vi "Climbing to Second Level.vi"(0 "close arms":bool, 1 "Second Preperation":bool, 2 "pull wire":bool, 3 "Open arms":bool, 4 "Abandon":bool) -> (5 "Prep 2":bool)   [LabVIEW 2012]
uses:
  <vilib>/Rock Robotics/WPI/PWM/Servo/WPI_ServoDeviceRef.ctl
  <vilib>/Rock Robotics/SystemInterfaces/Typedef/FPGA_TypedefDigitalModule.ctl
  <vilib>/Rock Robotics/SystemInterfaces/DIO/FPGA_DIOPWMChannel.ctl
  <vilib>/Rock Robotics/WPI/PWM/WPI_PWMDeadband.ctl
  <vilib>/Rock Robotics/WPI/MotorControl/WPI_MotorControlDeviceRef.ctl
  <vilib>/Rock Robotics/WPI/CAN/Jaguar/SubVIs/WPI_CANJaguar_ControlMode.ctl
  <vilib>/Rock Robotics/WPI/PWM/WPI_PWMTransform_ConPane.ctl
  BotStatus.vi
  Motors Values.vi
panel:
  out "cannenet vbus":dbl
  in  "Gyro Angle [degrees]":dbl
  in  "Analog Encoder Rotations [rotations]":dbl
  in  "distance of telescopit per one encoder rotation [m/rotations]":dbl
  in  "distance MAX of telescopit [m]":dbl
  in  "Telescopit Angle offset from horizon [degrees]":dbl
  in  "Telescopit set point Angle [degrees]":dbl
  in  "Start Climbing":bool
  out "telescopic vbus":dbl
  in  "Climbing":bool
  out "Telescopic Arms":dbl
  out "Canenet":dbl
  out "Climbing Enabled?":bool
  in  "Stop Climbing Override":bool
  in  "MotorControlDevRef 2":T1={"DeviceStatus"={"status"=FALSE, "code"=0, "source"=""}, "Type"=enum."PWM", "PWM"={"Digital Module"=enum."Digital Module 1", "PWM Channel"=enum."Invalid", "DeadBand"={"Name"="", "maxPositivePwm"=0, "minPositivePwm"=0, "centerPwm"=0, "maxNegativePwm"=0, "minNegativePwm"=0, "angularRange"=0}}, "CAN"={"Device Number"=0, "Control Mode"=enum."Percent VBus", "Semaphore"=refnum, "Max Vout"=12.0}, "Invert"=FALSE, "TransformRef"=refnum, "InvTransformRef"=refnum}
  in  "MotorControlDevRef 1":T1={"DeviceStatus"={"status"=FALSE, "code"=0, "source"=""}, "Type"=enum."PWM", "PWM"={"Digital Module"=enum."Digital Module 1", "PWM Channel"=enum."Invalid", "DeadBand"={"Name"="", "maxPositivePwm"=0, "minPositivePwm"=0, "centerPwm"=0, "maxNegativePwm"=0, "minNegativePwm"=0, "angularRange"=0}}, "CAN"={"Device Number"=0, "Control Mode"=enum."Percent VBus", "Semaphore"=refnum, "Max Vout"=12.0}, "Invert"=FALSE, "TransformRef"=refnum, "InvTransformRef"=refnum}
  in  "Climbing_ServoDeviceRef":T8={"DeviceStatus"={"status"=FALSE, "code"=0, "source"=""}, "Digital Module"=enum."Digital Module 1", "PWM Channel"=enum."Invalid", "DeadBand"={"Name"="", "maxPositivePwm"=0, "minPositivePwm"=0, "centerPwm"=0, "maxNegativePwm"=0, "minNegativePwm"=0, "angularRange"=0}}
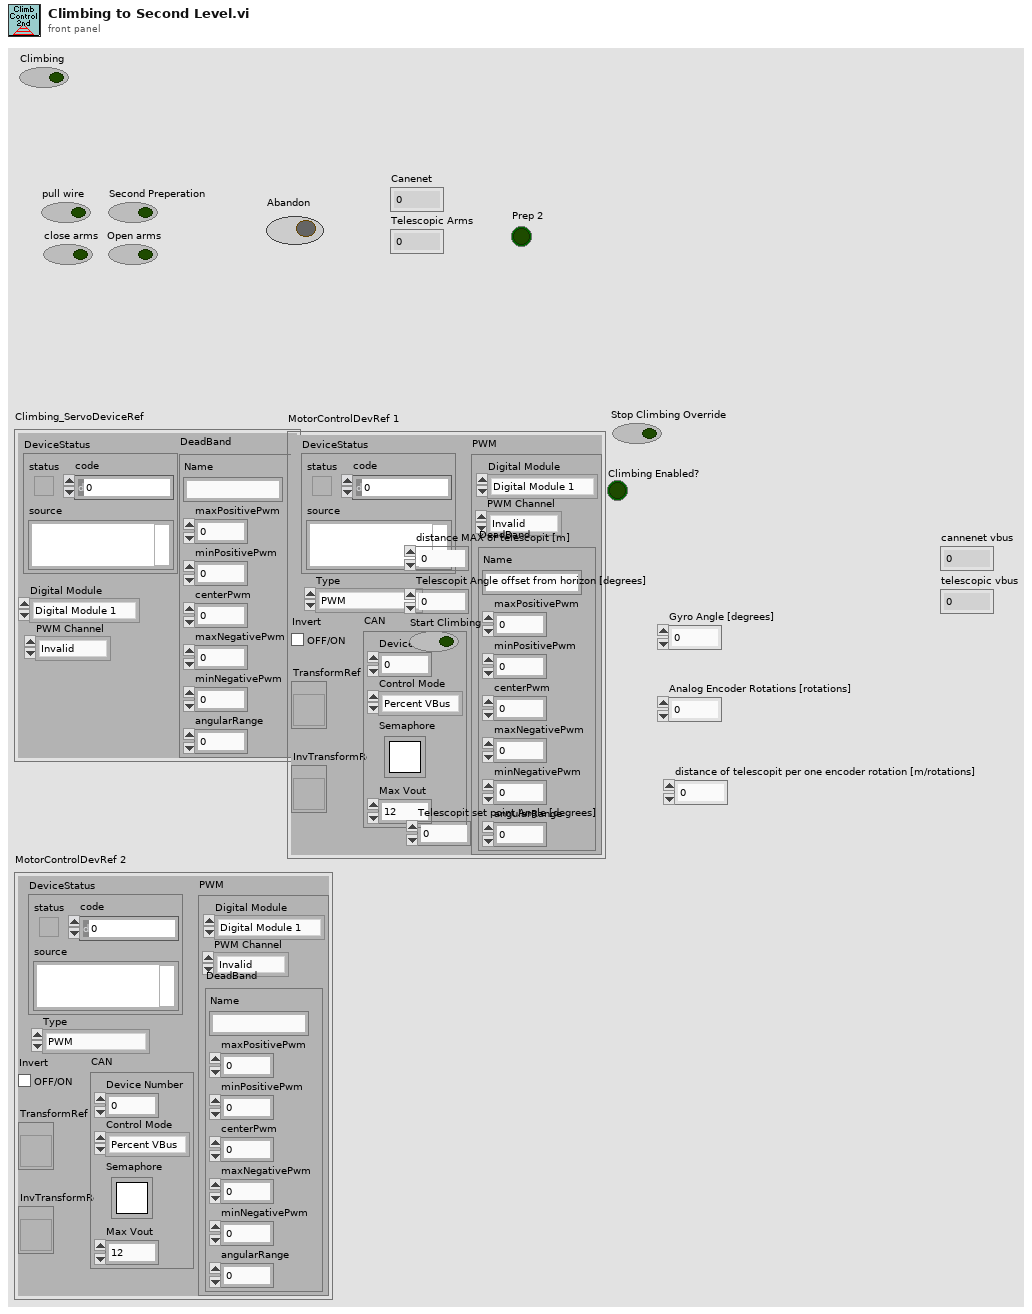
[diagram p1: front panel]
types:
  T1 = typedef "WPI_MotorControlDeviceRef.ctl" = cluster{"DeviceStatus":errorcluster, "Type":enum16{"PWM", "CAN"}, "PWM":cluster{"Digital Module":T2, "PWM Channel":T3, "DeadBand":T4}, "CAN":cluster{"Device Number":u8, "Control Mode":T5, "Semaphore":T6, "Max Vout":dbl}, "Invert":bool, "TransformRef":T7, "InvTransformRef":T7}
  T2 = typedef "FPGA_TypedefDigitalModule.ctl" = enum16{"Digital Module 1", "Digital Module 2"}
  T3 = typedef "FPGA_DIOPWMChannel.ctl" = enum8{"PWM 1", "PWM 2", "PWM 3", "PWM 4", "PWM 5", "PWM 6", "PWM 7", "PWM 8", "PWM 9", "PWM 10", "Invalid"}
  T4 = typedef "WPI_PWMDeadband.ctl" = cluster{"Name":string, "maxPositivePwm":i32, "minPositivePwm":i32, "centerPwm":i32, "maxNegativePwm":i32, "minNegativePwm":i32, "angularRange":u16}
  T5 = typedef "WPI_CANJaguar_ControlMode.ctl" = enum8{"Percent VBus", "Current", "Speed", "Position", "Voltage"}
  T6 = typedef "Semaphore RefNum" = refnum<k1>
  T7 = typedef "WPI_PWMTransform_ConPane.ctl" = refnum<vi>
  T8 = typedef "WPI_ServoDeviceRef.ctl" = cluster{"DeviceStatus":errorcluster, "Digital Module":T2, "PWM Channel":T3, "DeadBand":T4}
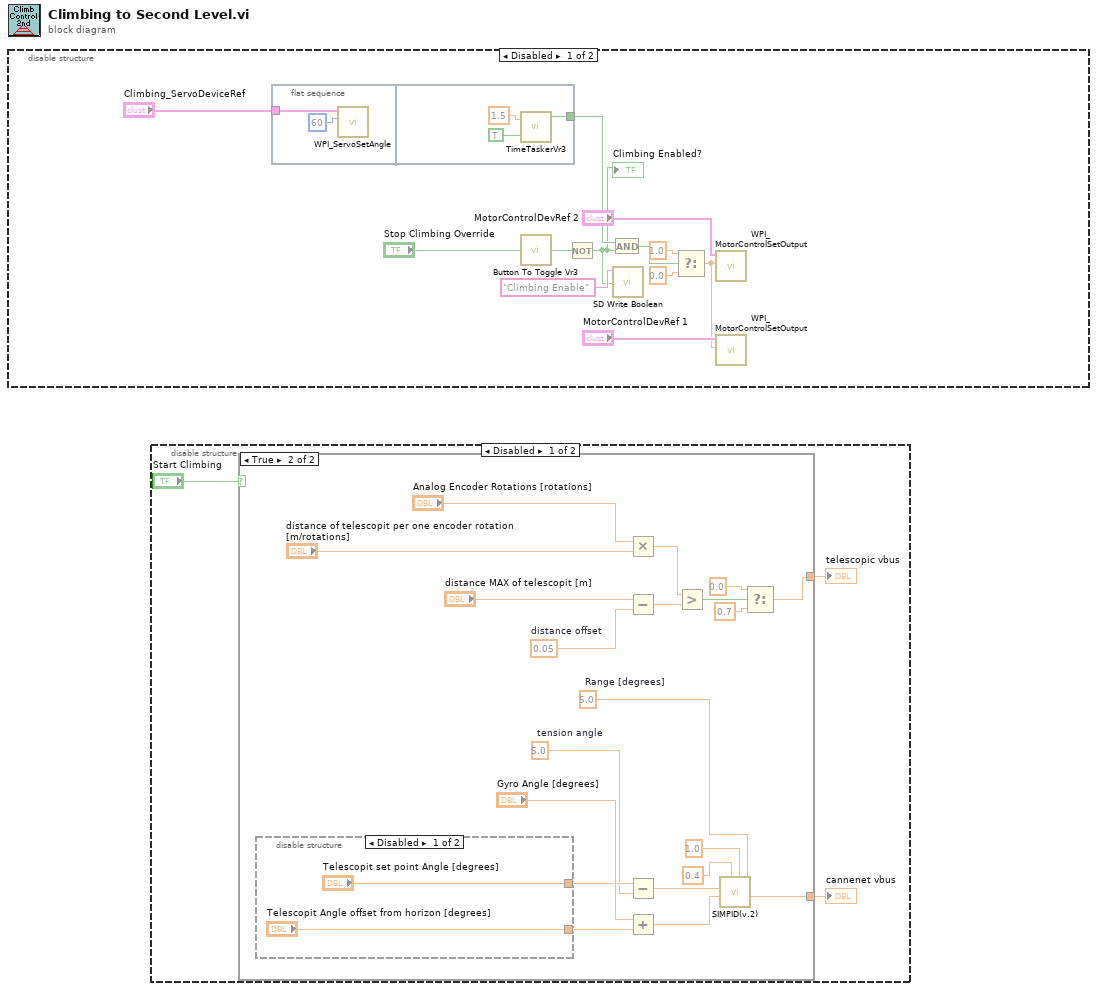
[diagram p0: block diagram]
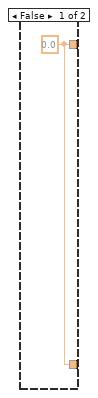
[diagram p2: hidden frame]
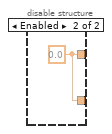
[diagram p3: hidden frame]
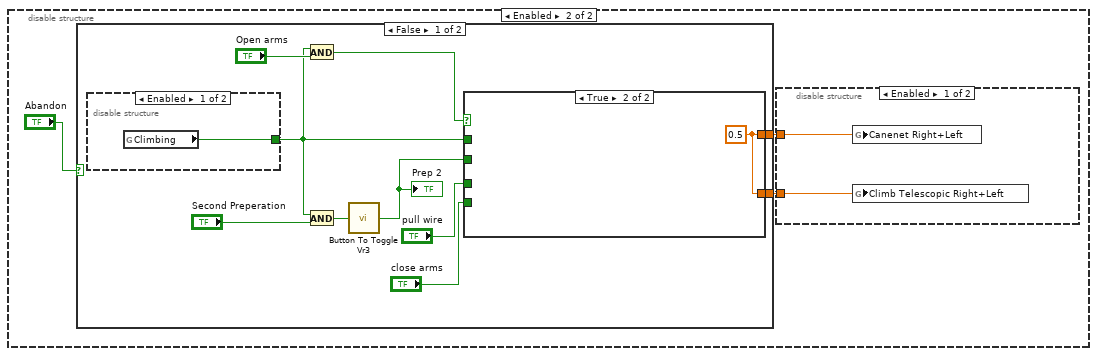
[diagram p5: hidden frame]
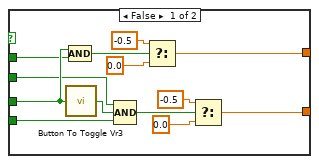
[diagram p6: hidden frame]
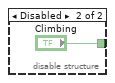
[diagram p7: hidden frame]
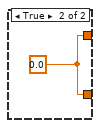
[diagram p8: hidden frame]
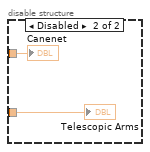
[diagram p9: hidden frame]
diagram:
  n1 = disable-structure shown="Disabled" {
    frame Disabled {
      n2 = flat-sequence {
        tunnel: "Climbing_ServoDeviceRef" -> [w14]
        tunnel: [w16] -> w7
        frame #0 {
          n3 = call <vilib>:"WPI_ServoSetAngle.vi"("Angle"=60, "ServoDeviceRef"=w14) -> ()  [unwired: 8 in, 2 out]
        }
        frame #1 {
          n4 = call "TimeTaskerVr3.vi"("Delay(sec)"=1.5, "Start Counting?"=TRUE) -> ("TimePast?"=w16:bool)  [unwired: 2 out]
        }
      }
      n5 = call "Button To Toggle Vr3.vi"("InValue"="Stop Climbing Override") -> ("Result"=w8:bool)
      n6 = Not(x=w8) -> (.not. x?=w1:bool)
      "Climbing Enabled?" <- w1
      n7 = And(x=w7, y=w1) -> (x .and. y?=w6:bool)
      n8 = call <vilib>:"SD Write Boolean.vi"("Boolean"=w1, "Name"="Climbing Enable") -> ()  [unwired: 8 in, 2 out]
      n9 = Select(t=1.0 ("Delay(sec)"), s=w6, f=0.0 ("Delay(sec)")) -> (s? t:f=w3:dbl)
      n10 = call <vilib>:"WPI_MotorControlSetOutput.vi"("Output"=w3, "MotorControlDevRef"="MotorControlDevRef 2") -> ()  [unwired: 7 in, 3 out]
      n11 = call <vilib>:"WPI_MotorControlSetOutput.vi"("Output"=w3, "MotorControlDevRef"="MotorControlDevRef 1") -> ()  [unwired: 7 in, 3 out]
    }
    frame Enabled {
      n12 = case shown="False" "Abandon" {
        tunnel: [w29 w47] -> w20
        tunnel: [w28 w47] -> w19
        frame False {
          n13 = disable-structure shown="Enabled" {
            disable-tunnel: [w45 "Climbing"] -> w26
            frame Enabled {
              n14 = global read "BotStatus.vi" "Climbing"() -> (w45:bool)
            }
            frame Disabled {
            }
          }
          n15 = And(x=w26, y="Open arms") -> (x .and. y?=w30:bool)
          n16 = And(x=w26, y="Second Preperation") -> (x .and. y?=w22:bool)
          n17 = call "Button To Toggle Vr3.vi"("InValue"=w22) -> ("Result"=w21:bool)
          "Prep 2" <- w21
          n18 = case shown="True" w30 {
            tunnel: "close arms" -> [w36 _]
            tunnel: "pull wire" -> [w33 _]
            tunnel: [w39 w44] -> w29
            tunnel: [w38 w44] -> w28
            tunnel: w26 -> [w32 _]
            tunnel: w21 -> [w31 _]
            frame False {
              n19 = call "Button To Toggle Vr3.vi"("InValue"=w33) -> ("Result"=w37:bool)
              n20 = Compound Arithmetic op=AND(w33, w32) -> (w34:bool)
              n21 = Compound Arithmetic op=AND(w31, w37, w36) -> (w35:bool)
              n22 = Select(t=-0.5, s=w34, f=0.0) -> (s? t:f=w39:dbl)
              n23 = Select(t=-0.5, s=w35, f=0.0) -> (s? t:f=w38:dbl)
            }
            frame True {
              w44 = 0.5 ("y")
            }
          }
        }
        frame True {
          w47 = 0.0
        }
      }
      n24 = disable-structure shown="Enabled" {
        disable-tunnel: w20 -> [w49 w51]
        disable-tunnel: w19 -> [w48 w50]
        frame Enabled {
          n25 = global write "Motors Values.vi" "Canenet Right+Left"(w49) -> ()
          n26 = global write "Motors Values.vi" "Climb Telescopic Right+Left"(w48) -> ()
        }
        frame Disabled {
          "Canenet" <- w51
          "Telescopic Arms" <- w50
        }
      }
    }
  }
  n27 = disable-structure shown="Disabled" {
    frame Disabled {
      n28 = case shown="True" "Start Climbing" {
        tunnel: [w55 w66] -> w52
        tunnel: [w55 w56] -> w54
        frame False {
          w55 = 0.0 ("result")
        }
        frame True {
          w57 = 0.05  # distance offset
          w64 = 5.0  # tension angle
          w67 = 5.0  # Range [degrees]
          n29 = disable-structure shown="Disabled" {
            disable-tunnel: ["Telescopit Angle offset from horizon [degrees]" w78] -> w73
            disable-tunnel: ["Telescopit set point Angle [degrees]" w78] -> w71
            frame Disabled {
            }
            frame Enabled {
              w78 = 0.0 ("Telescopit Angle offset from horizon [degrees]")
            }
          }
          n30 = Multiply(x="Analog Encoder Rotations [rotations]", y="distance of telescopit per one encoder rotation [m/rotations]") -> (x*y=w63:dbl)
          n31 = Subtract(x="distance MAX of telescopit [m]", y=w57) -> (x-y=w58:dbl)
          n32 = Subtract(x=w71, y=w64) -> (x-y=w65:dbl)
          n33 = Add(x="Gyro Angle [degrees]", y=w73) -> (x+y=w70:dbl)
          n34 = Greater?(x=w63, y=w58) -> (0:w61:bool)
          n35 = call "SIMPID(v.2).vi"("Range"=w67, "upper limit"=1.0, "lower limit"=0.4, "Current Point"=w70, "Set Point"=w65) -> ("result"=w66:dbl)  [unwired: 5 in, 1 out]
          n36 = Select(t=0.0, s=w61, f=0.7) -> (s? t:f=w56:dbl)
        }
      }
      "cannenet vbus" <- w52
      "telescopic vbus" <- w54
    }
    frame Enabled {
    }
  }
